vi "IEEE754-to-SGL_v1.vi"(11 "Input_U8":u8[](array[numeric])) -> (3 "Output_SGL":sgl=92.92 format="%.10f")   [LabVIEW 2017]
panel:
  out "Exponent":i32=6
  out "Mantissa":bool[](array[boolean])=[FALSE, TRUE, TRUE, TRUE, FALSE, FALSE, TRUE, TRUE, TRUE, FALSE, TRUE, FALSE, TRUE, TRUE, TRUE, FALSE, FALSE, FALSE, FALSE, TRUE, FALSE, TRUE, FALSE]
  out "Exponent":bool[](array[boolean])=[TRUE, FALSE, FALSE, FALSE, FALSE, TRUE, FALSE, TRUE]
  out "Sign":bool
  out "Mantissa":dbl=1.4518749713897705 format="%.8f"
  out "appended array 1D":bool[](array[boolean])
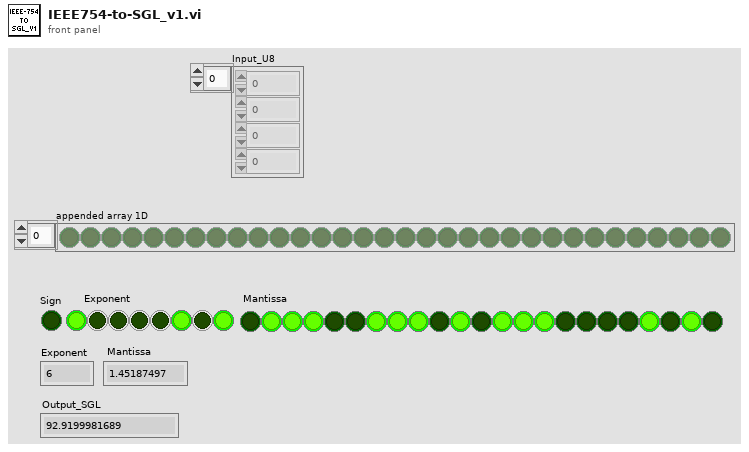
[diagram p1: front panel]
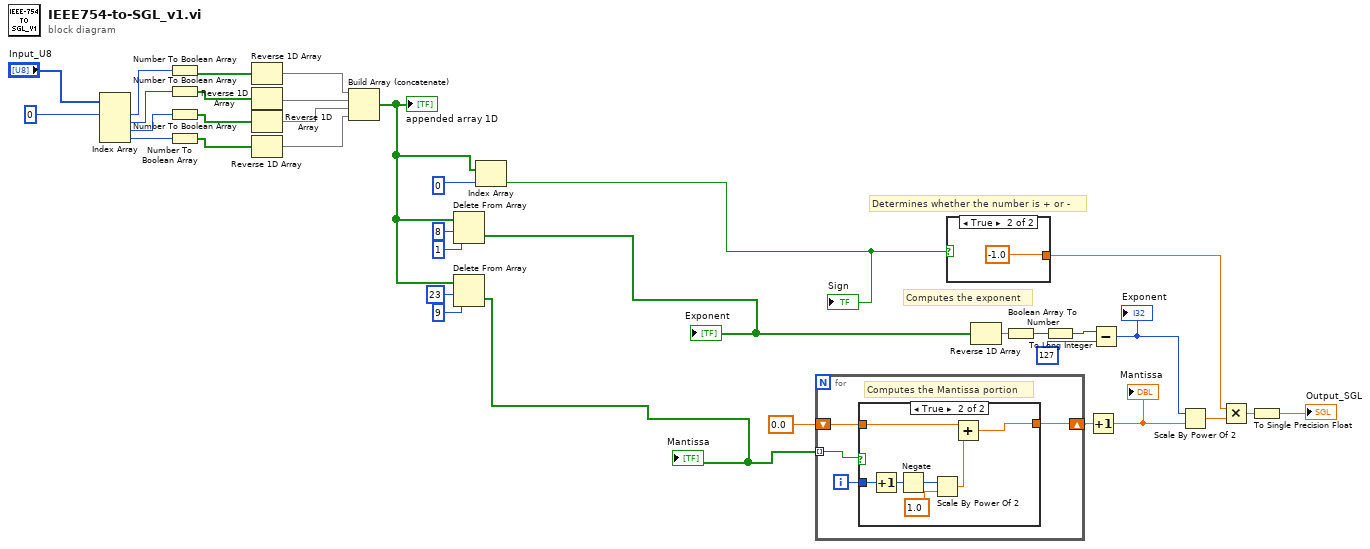
[diagram p0: block diagram]
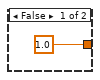
[diagram p2: hidden frame]
diagram:
  # "Computes the exponent"
  # "Determines whether the number is + or -"
  n1 = Index Array(array="Input_U8", index #1=0 ("index")) -> (element #1=w12:u8, element #2=w11:u8, element #3=w10:u8, element #4=w9:u8)  [unwired: 3 in]
  n2 = Number To Boolean Array(number=w12) -> (Boolean array=w7:bool[])
  n3 = Number To Boolean Array(number=w11) -> (Boolean array=w6:bool[])
  n4 = Number To Boolean Array(number=w10) -> (Boolean array=w5:bool[])
  n5 = Number To Boolean Array(number=w9) -> (Boolean array=w4:bool[])
  n6 = Reverse 1D Array(array=w7) -> (reversed array=w8:bool[])
  n7 = Reverse 1D Array(array=w6) -> (reversed array=w1:bool[])
  n8 = Reverse 1D Array(array=w5) -> (reversed array=w2:bool[])
  n9 = Reverse 1D Array(array=w4) -> (reversed array=w3:bool[])
  n10 = Build Array (concatenate)(w8, w1, w2, w3) -> (w17:bool[])
  "appended array 1D" <- w17
  n11 = Delete From Array(array=w17, length=8, index=1) -> (deleted portion=w19:bool[])  [unwired: 1 out]
  "Exponent" <- w19
  n12 = Delete From Array(array=w17, length=23, index=9) -> (deleted portion=w18:bool[])  [unwired: 1 out]
  "Mantissa" <- w18
  n13 = Index Array(array=w17, index=0) -> (element=w15:bool)
  "Sign" <- w15
  n14 = for {
    tunnel: w18 -> [w39] mode=indexing
    shift-right: [w36] -> w34
    shift-left: 0.0 -> [w37]
    i -> [w38]
    # "Computes the Mantissa portion"
    n15 = case shown="True" w39 {
      tunnel: w38 -> [_ w47]
      tunnel: w37 -> [w40 w43]
      tunnel: [w40 w41] -> w36
      frame False {
      }
      frame True {
        n16 = Increment(x=w47) -> (x+1=w46:i32)
        n17 = Negate(x=w46) -> (-x=w45:i32)
        n18 = Scale By Power Of 2(n=w45, x=1.0) -> (x*2^n=w42:dbl)
        n19 = Add(x=w43, y=w42) -> (x+y=w41:dbl)
      }
    }
  }
  n20 = case shown="True" w15 {
    tunnel: [1.0 -1.0] -> w28
    frame False {
    }
    frame True {
    }
  }
  n21 = Reverse 1D Array(array=w19) -> (reversed array=w30:bool[])
  n22 = Boolean Array To Number(Boolean array=w30) -> (number=w26:u32)
  n23 = To Long Integer(number=w26) -> (32bit integer=w25:i32)
  n24 = Increment(x=w34) -> (x+1=w32:dbl)
  "Mantissa" <- w32
  n25 = Subtract(x=w25, y=127) -> (x-y=w27:i32)
  "Exponent" <- w27
  n26 = Scale By Power Of 2(n=w27, x=w32) -> (x*2^n=w31:dbl)
  n27 = Multiply(x=w28, y=w31) -> (x*y=w29:dbl)
  n28 = To Single Precision Float(number=w29) -> (single precision float=→"Output_SGL":sgl)
